vi "Preview Stack.vi"(8 "error in (no error)":errorcluster, 11 "UPNCalculator in":refnum<class "UPNCalculator.lvclass">) -> (0 "error out":errorcluster, 2 "Stack":dbl[](array[numeric]), 3 "UPNCalculator out":refnum<class "UPNCalculator.lvclass">)   [LabVIEW 2016, in "UPNCalculator Actor.lvlib" / "UPNCalculator.lvclass"]
doc: "Returns the a preview of stack contents."
uses:
  UPNCalculator.lvclass
  UPNCalculator.lvclass/UPNCalculator.ctl
  Stack/Stack.lvclass
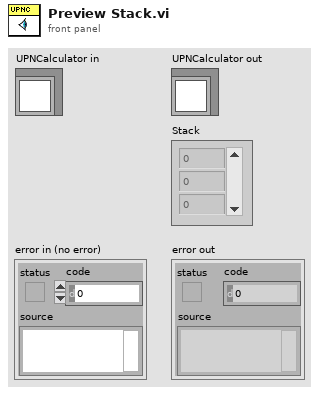
[diagram p1: front panel]
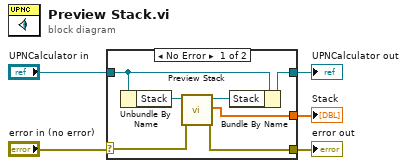
[diagram p0: block diagram]
diagram:
  n1 = case shown="No Error" "error in (no error)" {
    selector: "error in (no error)" -> [w11 w14]
    tunnel: [w10 w14] -> w4
    tunnel: [w7 w13] -> w2
    tunnel: "UPNCalculator in" -> [w8 w13]
    tunnel: [w9 _] -> w1
    frame No Error {
      n2 = Unbundle By Name(w8) -> ("Stack"=w12:refnum<class "Stack.lvclass">)
      n3 = call "Preview Stack.vi"("error in (no error)"=w11, "Stack in"=w12) -> ("error out"=w10:errorcluster, "Stack"=w9:dbl[], "Stack out"=w6:refnum<class "Stack.lvclass">)  [unwired: 7 in]
      n4 = Bundle By Name(cluster=w8, "Stack"=w6) -> (w7:refnum<class "UPNCalculator.lvclass">)
    }
    frame Error {
    }
  }
  "error out" <- w4
  "UPNCalculator out" <- w2
  "Stack" <- w1
